vi "Crossing within Limits.vi"(8 "error in (no error)":errorcluster, 9 "Limits":cluster{"Min":i64, "Max":i64}={"Min"=200000000000000, "Max"=400000000000000}, 10 "Vector 2":refnum<class "Vector.lvclass">, 11 "Vector In":refnum<class "Vector.lvclass">) -> (0 "error out":errorcluster, 1 "Coordinate":T1, 2 "Crossing within Limits?":bool)   [LabVIEW 2021, in "Vector.lvclass"]
uses:
  Vector.lvclass
  High Res Arithmetic/Rational Number.lvclass
  Vector.lvclass/Vector.ctl
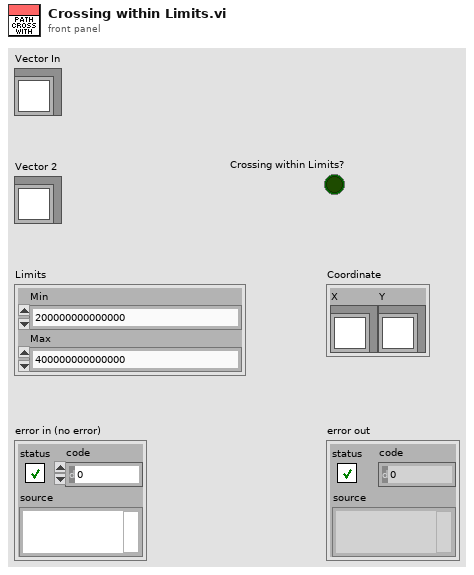
[diagram p1: front panel]
types:
  T1 = cluster{"X":refnum<class "Rational Number.lvclass">, "Y":refnum<class "Rational Number.lvclass">}
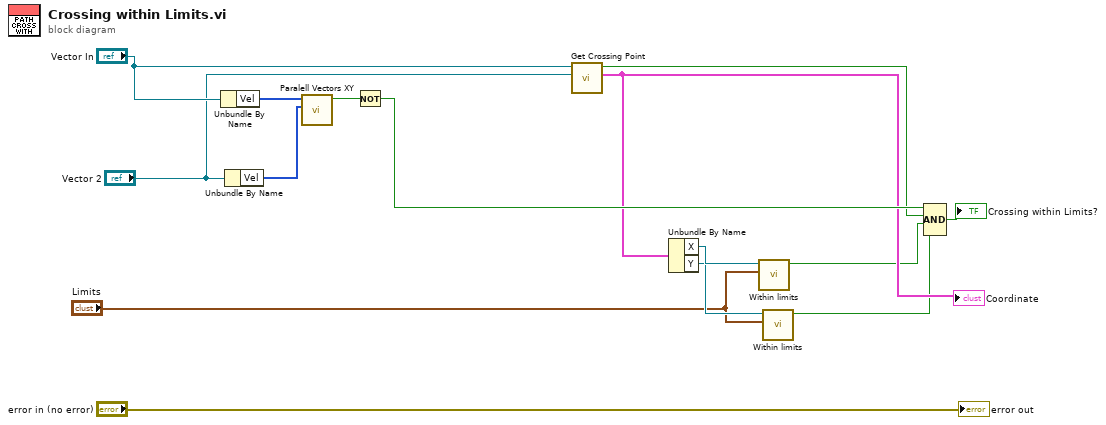
[diagram p0: block diagram]
diagram:
  n1 = Unbundle By Name("Vector In") -> ("Vel"=w13:i64[])
  n2 = Unbundle By Name("Vector 2") -> ("Vel"=w12:i64[])
  n3 = call "Paralell Vectors XY.vi"("Vector 2"=w12, "Vector 1"=w13) -> ("Boolean"=w10:bool)  [unwired: 9 in]
  n4 = Not(x=w10) -> (.not. x?=w11:bool)
  n5 = call "Get Crossing Point.vi"("Vector 2"="Vector 2", "Vector in"="Vector In") -> ("Coordinate"=w6:T1, "In Future?"=w7:bool)  [unwired: 8 in]
  "Coordinate" <- w6
  n6 = Unbundle By Name(w6) -> ("X"=w5:refnum<class "Rational Number.lvclass">, "Y"=w3:refnum<class "Rational Number.lvclass">)
  n7 = call "Within limits.vi"("Limits"="Limits", "Rational Number in"=w5) -> ("In Limits?"=w4:bool)  [unwired: 9 in]
  n8 = call "Within limits.vi"("Limits"="Limits", "Rational Number in"=w3) -> ("In Limits?"=w1:bool)  [unwired: 9 in]
  n9 = Compound Arithmetic op=AND(w11, w7, w4, w1) -> (→"Crossing within Limits?":bool)
  "error out" <- "error in (no error)"
